vi "Tabla_multiplicar.vi"() -> ()   [LabVIEW 2020]
panel:
  out "TABLA DE MULTIPLICAR":dbl[][](array[numeric])
  out "resultado":dbl
  in  "posicion\nvertical":i32
  in  "posicion \nhorizontal":i32
  in  "n de columnas":i32
  in  "n de renglones":i32
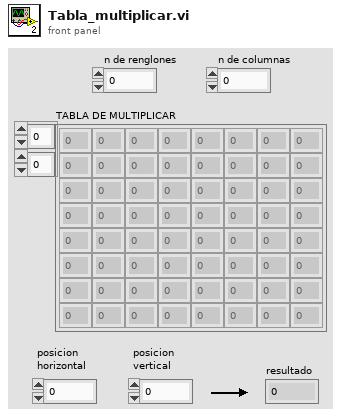
[diagram p1: front panel]
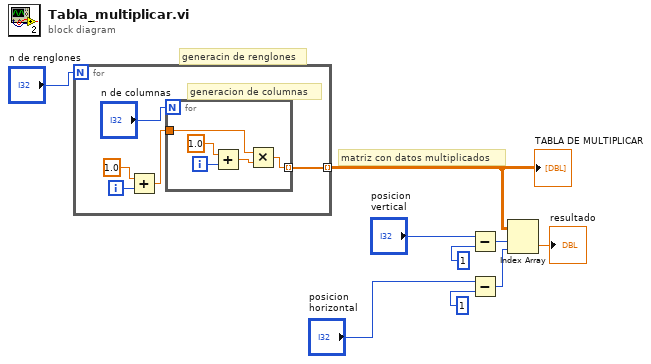
[diagram p0: block diagram]
diagram:
  # "matriz con datos multiplicados"
  # "generacin de renglones"
  n1 = for {
    N: "n de renglones" -> [_]
    tunnel: [w10] -> w8 mode=indexing
    i -> [w13]
    # "generacion de columnas"
    n2 = Add(x=1.0, y=w13) -> (x+y=w11:dbl)
    n3 = for {
      N: "n de columnas" -> [_]
      tunnel: w11 -> [w17]
      tunnel: [w15] -> w10 mode=indexing
      i -> [w18]
      n4 = Add(x=1.0, y=w18) -> (x+y=w16:dbl)
      n5 = Multiply(x=w17, y=w16) -> (x*y=w15:dbl)
    }
  }
  "TABLA DE MULTIPLICAR" <- w8
  n6 = Subtract(x="posicion\nvertical", y=1) -> (x-y=w2:i32)
  n7 = Subtract(x="posicion \nhorizontal", y=1) -> (x-y=w5:i32)
  n8 = Index Array(array=w8, index (row)=w2, index (col)=w5) -> (element=→"resultado":dbl)
